vi "Headers+String Arrays to SS File v3.vi"(5 "Header":string[][](array[string]), 6 "2d Data String Array":string[][](array[string]), 7 "1d Data String Array":string[](array[string]), 8 "error in":errorcluster, 9 "File Name":string, 10 "File Location":T2={"Log directory type"=1, "Rel Log Path"="LeakTemp"} {"Log directory type" items=["User Home"=0, "User Desktop"=1, "User Documents"=2, "User Application Data"=3, "User Preferences"=4, "User Temporary"=5, "Public Documents"=6, "Public Application Data"=7, "Public Preferences"=8, "Public Cache"=13, "System Core Libraries"=9, "System Installed Libraries"=10, "Application Files"=11, "Boot Volume Root"=12]}, 11 "Dir Path":path) -> (0 "error out":errorcluster, 2 "Actual file path":path)   [LabVIEW 2020]
uses:
  System Directory Type.ctl
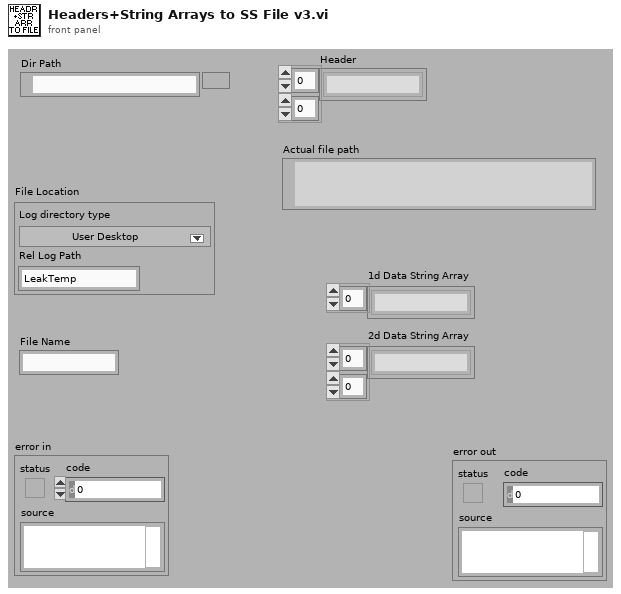
[diagram p1: front panel]
types:
  T1 = typedef "System Directory Type.ctl" = i32
  T2 = cluster{"Log directory type":T1, "Rel Log Path":string}
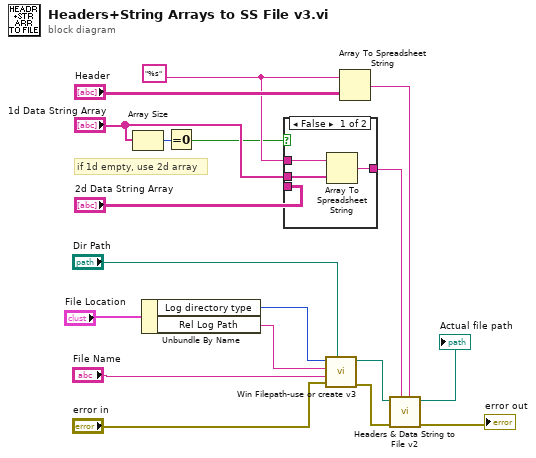
[diagram p0: block diagram]
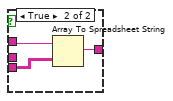
[diagram p2: hidden frame]
diagram:
  w16 = "%s" ("delimiter (Tab)")
  # "if 1d empty, use 2d array"
  n1 = Array Size(array="1d Data String Array") -> (size(s)=w13:i32)
  n2 = Unbundle By Name("File Location") -> ("Log directory type"=w3:T1, "Rel Log Path"=w2:string)
  n3 = Equal To 0?(x=w13) -> (x = 0?=w12:bool)
  n4 = case shown="False" w12 {
    tunnel: w16 -> [w21 w24]
    tunnel: [w20 w22] -> w10
    tunnel: "1d Data String Array" -> [w19 _]
    tunnel: "2d Data String Array" -> [_ w23]
    frame False {
      n5 = Array To Spreadsheet String(array=w19, 3:w21) -> (spreadsheet string=w20:string)  [unwired: 1 in]
    }
    frame True {
      n6 = Array To Spreadsheet String(array=w23, 3:w24) -> (spreadsheet string=w22:string)  [unwired: 1 in]
    }
  }
  n7 = call "Win Filepath-use or create v3.vi"("Dir Path"="Dir Path", "error in"="error in", "File Name"="File Name", "Subdir"=w2, "Win Directory Type"=w3) -> ("error out"=w8:errorcluster, "Filepath"=w1:path)  [unwired: 3 in]
  n8 = Array To Spreadsheet String(array="Header", 3:w16) -> (spreadsheet string=w9:string)  [unwired: 1 in]
  n9 = call "Headers & Data String to File v2.vi"("Header String"=w9, "Data Line String"=w10, "error in (no error)"=w8, "File Path"=w1) -> ("error out"=→"error out":errorcluster, "Path Out"=→"Actual file path":path)  [unwired: 4 in]
